vi "App Tag.vi"(8 "错误输入":errorcluster, 9 "Value":variant, 10 "Mode":T1(ring), 11 "Tag Name":string) -> (0 "错误输出":errorcluster, 3 "Old Value":variant)   [LabVIEW 2012, in "Application.lvlib"]
uses:
  Application.lvlib
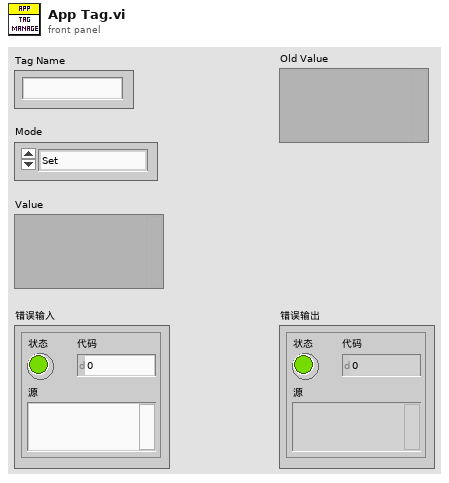
[diagram p1: front panel]
types:
  T1 = enum16{"Set", "Get", "Remove Tag", "Remove All Tags"}
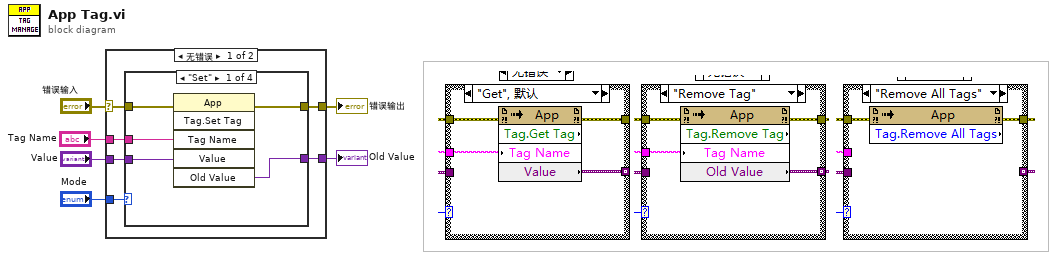
[diagram p0: block diagram]
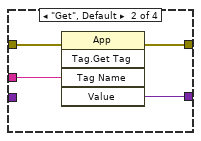
[diagram p2: hidden frame]
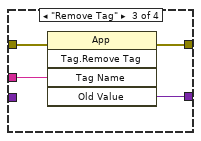
[diagram p3: hidden frame]
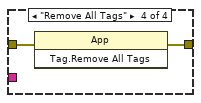
[diagram p4: hidden frame]
diagram:
  n1 = case shown="无错误" "错误输入" {
    selector: "错误输入" -> [w10 w28]
    tunnel: [w9 w28] -> w5
    tunnel: "Mode" -> [w12 _]
    tunnel: "Tag Name" -> [w11 _]
    tunnel: [w8 _] -> w2
    tunnel: "Value" -> [w7 _]
    frame No Error {
      n2 = case shown="\"Set\"" w12 {
        tunnel: w11 -> [w14 w21 w23 _]
        tunnel: w10 -> [w17 w20 w25 w27]
        tunnel: [w16 w19 w24 w26] -> w9
        tunnel: [w15 w18 w22 _] -> w8
        tunnel: w7 -> [w13 _ _ _]
        frame "Set" {
          n3 = invoke class="App" method="Tag.Set Tag"(error in=w17, "Tag Name"=w14, "Value"=w13) -> (error out=w16:errorcluster, "Old Value"=w15:variant)  [unwired: 3 in, 4 out]
        }
        frame "Get", Default {
          n4 = invoke class="App" method="Tag.Get Tag"(error in=w20, "Tag Name"=w21) -> (error out=w19:errorcluster, "Value"=w18:variant)  [unwired: 3 in, 3 out]
        }
        frame "Remove Tag" {
          n5 = invoke class="App" method="Tag.Remove Tag"(error in=w25, "Tag Name"=w23) -> (error out=w24:errorcluster, "Old Value"=w22:variant)  [unwired: 3 in, 3 out]
        }
        frame "Remove All Tags" {
          n6 = invoke class="App" method="Tag.Remove All Tags"(error in=w27) -> (error out=w26:errorcluster)  [unwired: 2 in, 2 out]
        }
      }
    }
    frame Error {
    }
  }
  "错误输出" <- w5
  "Old Value" <- w2
